vi "VariableStorage.vi"(9 "menu":enum16{"set", "get", "delete"}(ring), 10 "var name":string, 11 "Data":dbl) -> (3 "Data Out":dbl)   [LabVIEW 2011]
doc: "Sets a reference into a registry, gets a reference from a registry, or deletes a reference from a registry. The reference is accessed by name, and can be given any unique name.\n\nThis software is licensed. Open the labview\\readme\\WPI Robotics Library Open Source License.txt file for more information."
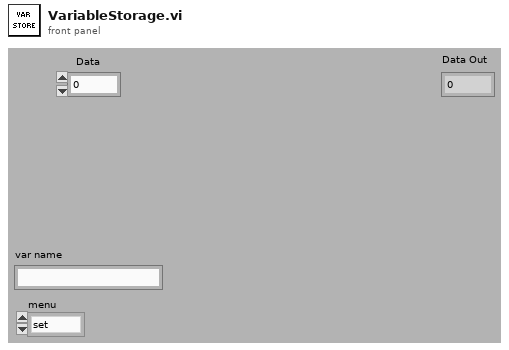
[diagram p1: front panel]
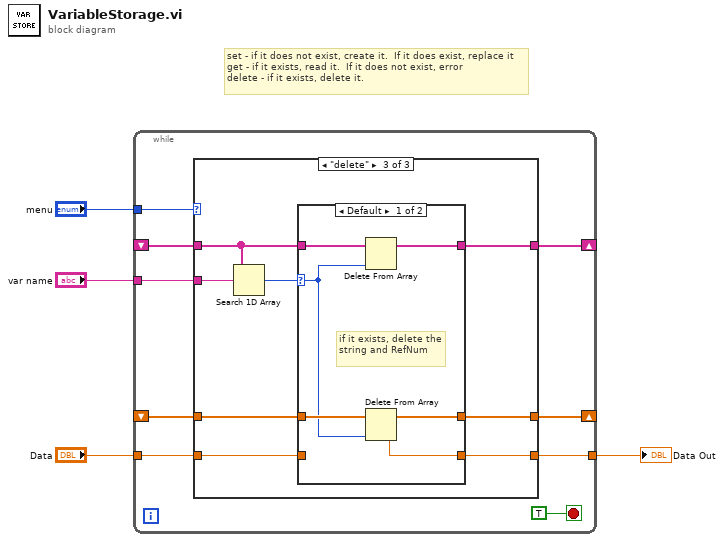
[diagram p0: block diagram]
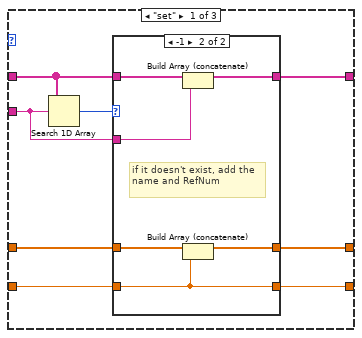
[diagram p2: hidden frame]
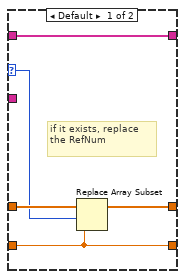
[diagram p3: hidden frame]
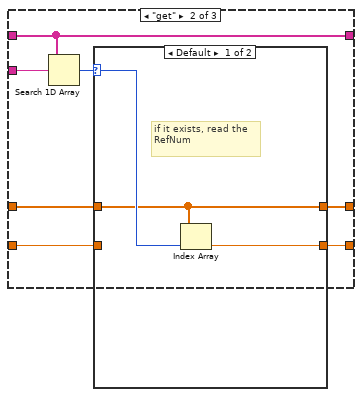
[diagram p4: hidden frame]
diagram:
  # "set - if it does not exist, create it.  If it does exist, replace it\nget - if it exists, read it.  If it does not exist, error\ndelete - if it exists, delete it."
  n1 = while {
    tunnel: "Data" -> [w13]
    tunnel: "var name" -> [w6]
    shift-right: [w12] -> _
    shift-left: _ -> [w11]
    tunnel: [w10] -> w2
    tunnel: "menu" -> [w9]
    shift-right: [w8] -> _
    shift-left: _ -> [w7]
    stop <- TRUE stop-if-true
    n2 = case shown="\"delete\"" w9 {
      tunnel: w13 -> [w16 w36 w46]
      tunnel: [w15 w35 w45] -> w12
      tunnel: w11 -> [w17 w37 w47]
      tunnel: [w14 w34 w44] -> w10
      tunnel: [w21 w33 w51] -> w8
      tunnel: w7 -> [w20 w33 w50]
      tunnel: w6 -> [w18 w38 w48]
      frame "set" {
        n3 = Search 1D Array(1D array=w20, element=w18) -> (index of element=w19:i32)  [unwired: 1 out]
        n4 = case shown="-1" w19 {
          selector: w19 -> [w24 _]
          tunnel: [w26 w32] -> w21
          tunnel: w20 -> [w26 w31]
          tunnel: w18 -> [_ w30]
          tunnel: w17 -> [w25 w29]
          tunnel: w16 -> [w22 w27]
          tunnel: [w23 w28] -> w15
          tunnel: [w22 w27] -> w14
          frame Default {
            # "if it exists, replace the RefNum"
            n5 = Replace Array Subset(array=w25, new element=w22, index=w24) -> (w23:dbl[])
          }
          frame -1 {
            # "if it doesn't exist, add the name and RefNum"
            n6 = Build Array (concatenate)(w31, w30) -> (w32:string[])
            n7 = Build Array (concatenate)(w29, w27) -> (w28:dbl[])
          }
        }
      }
      frame "get" {
        n8 = Search 1D Array(1D array=w33, element=w38) -> (index of element=w39:i32)  [unwired: 1 out]
        n9 = case shown="Default" w39 {
          selector: w39 -> [w42 _]
          tunnel: w37 -> [w40 w43]
          tunnel: w36 -> [_ _]
          tunnel: [w40 w43] -> w35
          tunnel: [w41 _] -> w34
          frame Default {
            # "if it exists, read the RefNum"
            n10 = Index Array(array=w40, index=w42) -> (element=w41:dbl)
          }
          frame -1 {
            # "if it doesn't exist, return default and set an error"
          }
        }
      }
      frame "delete" {
        n11 = Search 1D Array(1D array=w50, element=w48) -> (index of element=w49:i32)  [unwired: 1 out]
        n12 = case shown="Default" w49 {
          selector: w49 -> [w52 _]
          tunnel: [w53 w59] -> w51
          tunnel: w50 -> [w54 w59]
          tunnel: w47 -> [w57 w58]
          tunnel: w46 -> [_ w60]
          tunnel: [w56 w58] -> w45
          tunnel: [w55 w60] -> w44
          frame Default {
            # "if it exists, delete the string and RefNum"
            n13 = Delete From Array(array=w54, index=w52) -> (array with subset deleted=w53:string[])  [unwired: 1 in, 1 out]
            n14 = Delete From Array(array=w57, index=w52) -> (deleted portion=w55:dbl, array with subset deleted=w56:dbl[])  [unwired: 1 in]
          }
          frame -1 {
            # "if it doesn't exist, do nothing"
          }
        }
      }
    }
  }
  "Data Out" <- w2
